vi "EletoMatr-no trigger.vi"(0 "Input Array":dbl[][](array[numeric]), 5 "Input":dbl, 9 "In Row":i32, 11 "In Column":i32, 12 "Input Direction":bool=TRUE) -> (4 "Out Array":dbl[][](array[numeric]), 6 "Output Direction":bool=TRUE, 10 "Out Row":i32, 15 "Out Column":i32)   [LabVIEW 2018]
uses:
  <vilib>/Analysis/Matrix/Numeric/Conversions/Matrix To Array - RM.vi
  <vilib>/Analysis/Matrix/NI_Matrix.lvlib
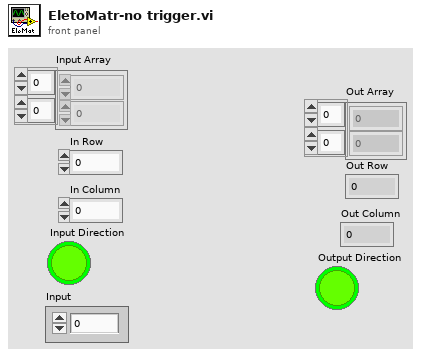
[diagram p1: front panel]
types:
  T1 = typedef "NI_Matrix.lvlib/RealMatrix.ctl" = dbl[][]
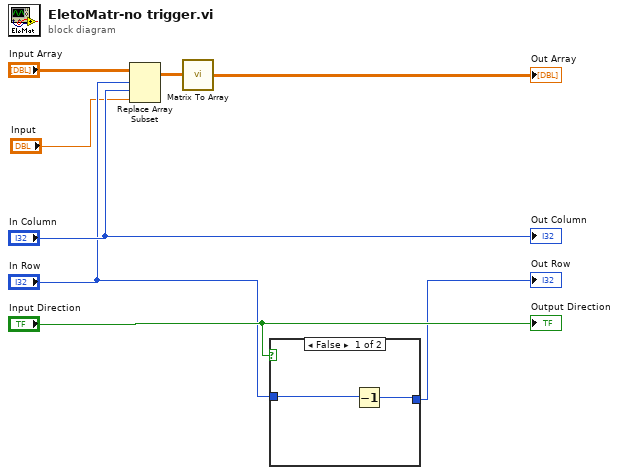
[diagram p0: block diagram]
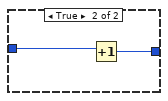
[diagram p2: hidden frame]
diagram:
  n1 = Replace Array Subset(array="Input Array", new element="Input", index (row)="In Row", index (col)="In Column") -> (w2:T1)
  n2 = call-poly <vilib>:"Matrix To Array.vi"("Real Matrix"=w2) -> ("Real 2D Array"=→"Out Array":dbl[][])
  n3 = case shown="False" "Input Direction" {
    tunnel: [w10 w12] -> w7
    tunnel: "In Row" -> [w9 w11]
    frame False {
      n4 = Decrement(x=w9) -> (x-1=w10:i32)
    }
    frame True {
      n5 = Increment(x=w11) -> (x+1=w12:i32)
    }
  }
  "Out Row" <- w7
  "Out Column" <- "In Column"
  "Output Direction" <- "Input Direction"
